vi "OceanOptics_TriggerPlayground_2.vi"() -> ()   [LabVIEW 2016]
uses:
  Maya2000 Typedefs/Maya2000 basic info.ctl
  <vilib>/Platform/TimedLoop/XDataNode/timing_clust.ctl
  <vilib>/Platform/TimedLoop/XDataNode/nitl_modes.ctl
  <vilib>/Platform/TimedLoop/XDataNode/wakeup.ctl
  C:/Program Files/Ocean Optics/OmniDriver/OOI_HOME/NETOmniDriver-NET40.dll
  Program Files/Ocean Optics/OmniDriver/OOI_HOME/NETOmniDriver-NET40.dll
  <vilib>/platform/TimedLoop/XDataNode/XDataNode.xnode
  <vilib>/Platform/TimedLoop/XDataNode/XDNodeRunTimeDep.lvlib
panel:
  out "spectrum":cluster{"Y":dbl[], "Y":dbl[]}[](graph)
  out "getExternalTriggerMode":i32
  in  "Trigger mode":i32
  out "isEnableBuffer":i32
  out "getBufferCapacity":i32
  in  "setBufferCoapacity":i32
  out "isFeatureSupportedDataBuffer":i16
  in  "clear":bool
  out "error Loop":errorcluster caption="error out"
  out "getExternalTriggerDelayIncrement":i32
  out "read":bool
  out "getBufferCapacity in Loop":i32
  out "getNumberOfElements before readout":i32
  out "status":bool
  out "error out":errorcluster
  out "this maya":T1={"This instruments index"=0, "Name+SerialNumber"="MayaPro2000:MAYP111403", "Number Dark pixels"=8, "NumberOfPixels\nper spectrum"=2068, "NumberOf Maya2000 instrm."=2, "MaximumIntegrationTime\n[us]"=1600000000, "MinimumIntegrationTime\n[us]"=7200}
  in  "stop":bool
  in  "integration time [us]":i32=100000
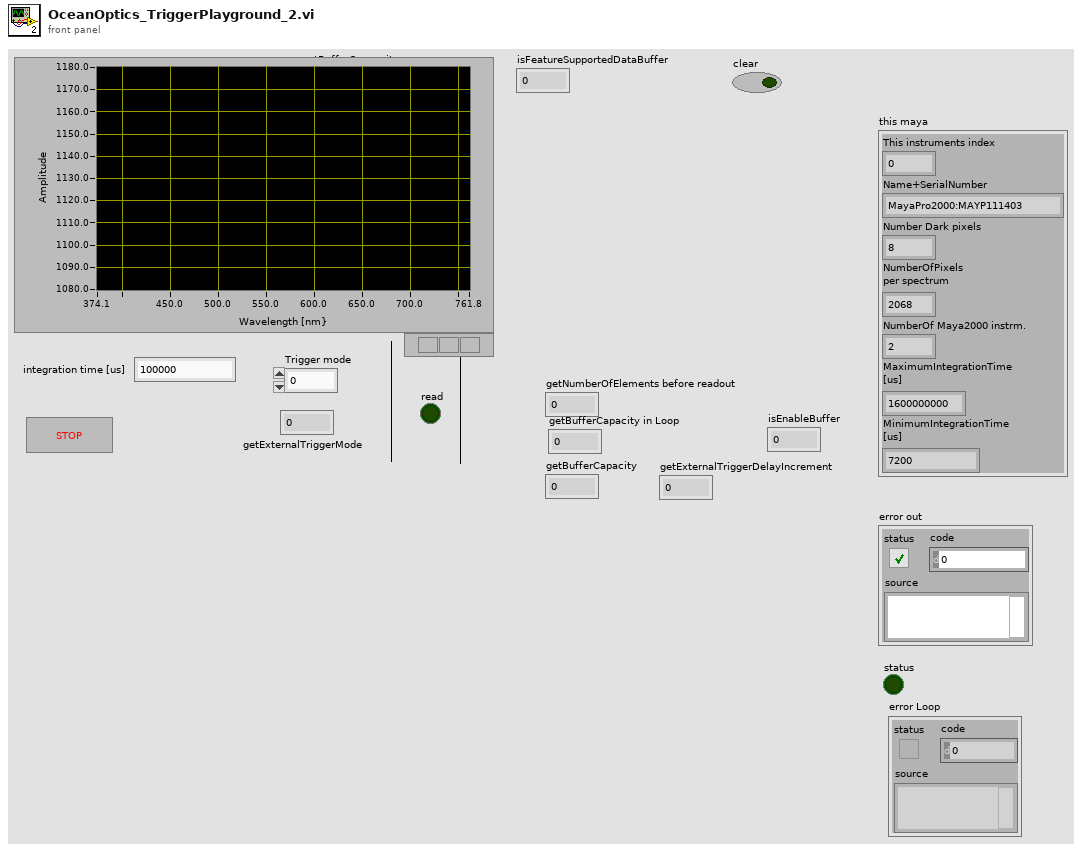
[diagram p1: front panel]
types:
  T1 = typedef "Maya2000 basic info.ctl" = cluster{"This instruments index":i32, "Name+SerialNumber":string, "Number Dark pixels":i32, "NumberOfPixels\nper spectrum":i32, "NumberOf Maya2000 instrm.":i32, "MaximumIntegrationTime\n[us]":i32, "MinimumIntegrationTime\n[us]":i32}
  T2 = typedef "XDNodeRunTimeDep.lvlib/timing_clust.ctl" = cluster{"Expected End [f-1]":u64, "Actual End [f-1]":u64, "Finished Late? [f-1]":bool, "Expected End [i-1]":u64, "Actual End [i-1]":u64, "Finished Late? [i-1]":bool, "Expected Start [i]":u64, "Actual Start [i]":u64, "Expected Start [f]":u64, "Actual Start [f]":u64, "Source Name":string, "Structure Name":string, "Period":i64, "Deadline":i64, "Offset":i64, "Start":i64, "Priority":i32, "Timeout":i32, "Mode":T3, "Wakeup Reason":T4, "Error":errorcluster, "Source Type":string, "Secondary Source Type":string, "Global End Time":u64, "Global Start Time":u64, "Frame Duration":u64, "Iteration Duration":u64, "Assigned CPU":i32, "I/O Scan Engine Mode":u32}
  T3 = typedef "XDNodeRunTimeDep.lvlib/nitl_modes.ctl" = enum32{"No Change", "Process missed periods, maintain original phase", "Discard missed periods, maintain original phase", "Process missed periods, ignore original phase", "Discard missed periods, ignore original phase"}
  T4 = typedef "XDNodeRunTimeDep.lvlib/wakeup.ctl" = enum32{"Normal", "Aborted", "Asynchronous wakeup", "Timing source error", "Timed loop error", "Timeout"}
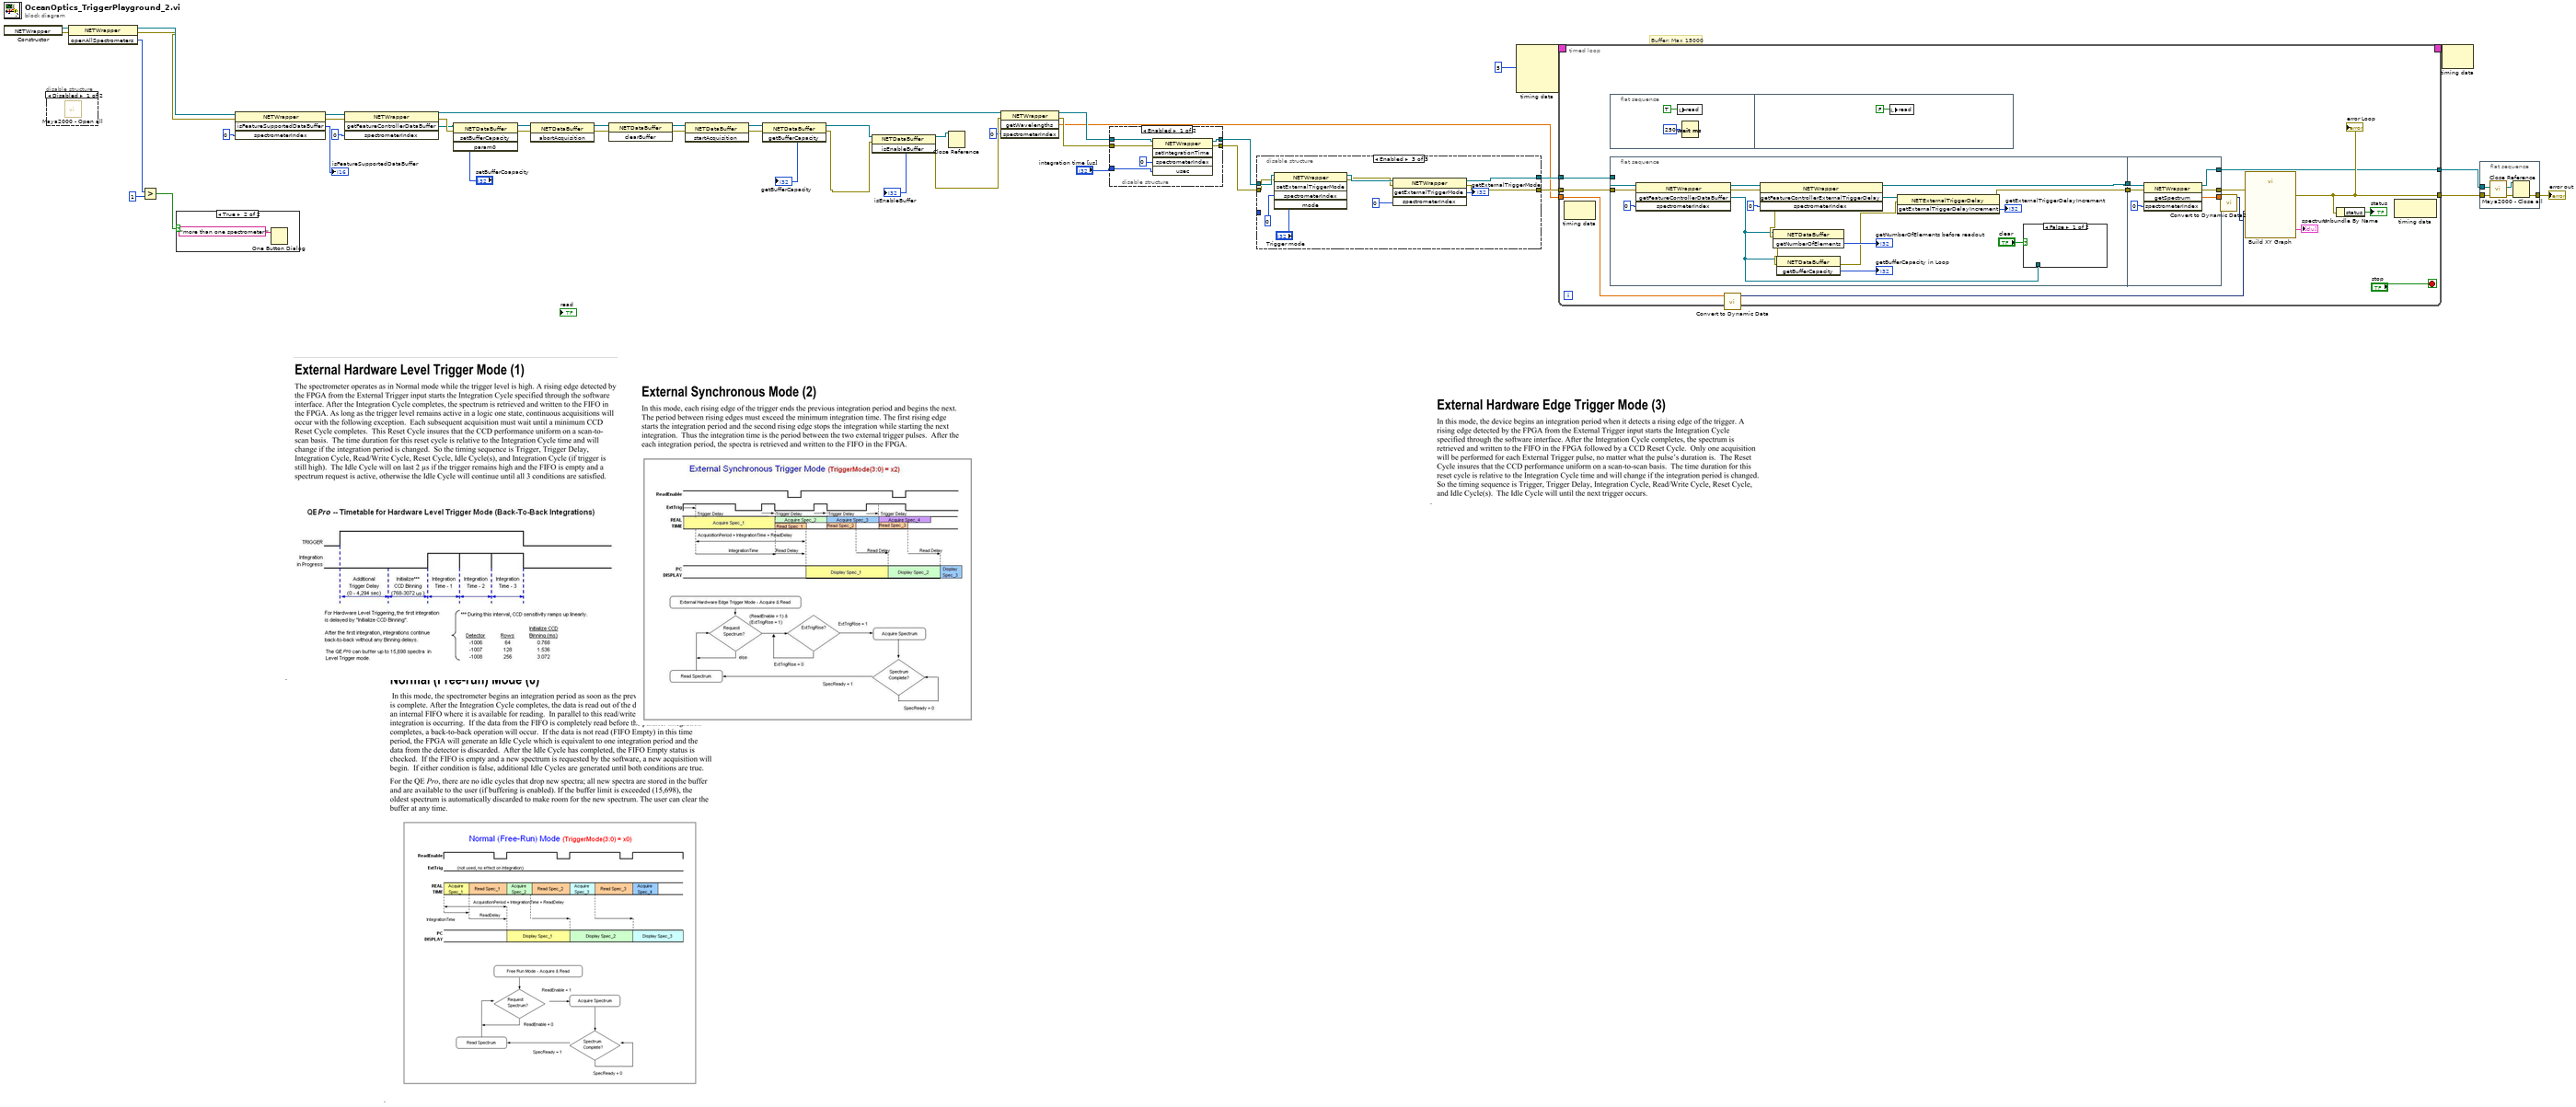
[diagram p0: block diagram]
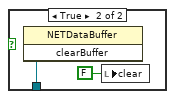
[diagram p3: hidden frame]
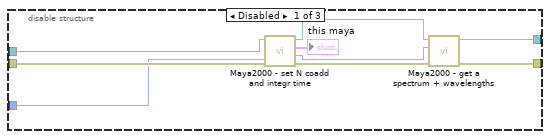
[diagram p4: hidden frame]
diagram:
  # "Buffer: Max 15000"
  n1 = constructor class="NETWrapper"() -> (reference out=w17:refnum<k24>, error out=w16:errorcluster)  [unwired: 3 in, 1 out]
  n2 = disable-structure shown="Disabled" {
    frame Disabled {
      n3 = call "Maya2000 - Open all.vi"() -> ()  [unwired: 9 in, 3 out]
    }
    frame Enabled {
    }
  }
  n4 = invoke class="NETWrapper" method="openAllSpectrometers"(reference=w17, error in=w16) -> (reference out=w15:refnum<k24>, error out=w14:errorcluster, "openAllSpectrometers"=w12:i32)  [unwired: 1 in]
  n5 = Greater?(x=w12, y=1) -> (0:w13:bool)
  n6 = case shown="True" w13 {
    frame False {
    }
    frame True {
      n7 = One Button Dialog(message="more than one spectrometer!") -> ()  [unwired: 1 in, 1 out]
    }
  }
  n8 = invoke class="NETWrapper" method="isFeatureSupportedDataBuffer"(reference=w15, error in=w14, "spectrometerIndex"=0) -> (reference out=w34:refnum<k24>, error out=w33:errorcluster, "isFeatureSupportedDataBuffer"=→"isFeatureSupportedDataBuffer":i16)  [unwired: 1 in, 1 out]
  n9 = invoke class="NETWrapper" method="getFeatureControllerDataBuffer"(reference=w34, error in=w33, "spectrometerIndex"=0) -> (reference out=w9:refnum<k24>, error out=w37:errorcluster, "getFeatureControllerDataBuffer"=w10:refnum<k24>)  [unwired: 1 in, 1 out]
  n10 = invoke class="NETDataBuffer" method="setBufferCapacity"(reference=w10, error in=w37, "param0"="setBufferCoapacity") -> (reference out=w22:refnum<k24>, error out=w31:errorcluster)  [unwired: 1 in, 2 out]
  n11 = invoke class="NETDataBuffer" method="abortAcquisition"(reference=w22, error in=w31) -> (reference out=w29:refnum<k24>, error out=w28:errorcluster)  [unwired: 1 in, 1 out]
  n12 = invoke class="NETDataBuffer" method="clearBuffer"(reference=w29, error in=w28) -> (reference out=w27:refnum<k24>, error out=w26:errorcluster)  [unwired: 1 in, 1 out]
  n13 = invoke class="NETDataBuffer" method="startAcquisition"(reference=w27, error in=w26) -> (reference out=w25:refnum<k24>, error out=w24:errorcluster)  [unwired: 1 in, 1 out]
  n14 = invoke class="NETDataBuffer" method="getBufferCapacity"(reference=w25, error in=w24) -> (reference out=w21:refnum<k24>, error out=w20:errorcluster, "getBufferCapacity"=→"getBufferCapacity":i32)  [unwired: 1 in]
  n15 = invoke class="NETDataBuffer" method="isEnableBuffer"(reference=w21, error in=w20) -> (reference out=w18:refnum<k24>, error out=w8:errorcluster, "isEnableBuffer"=→"isEnableBuffer":i16)  [unwired: 1 in]
  n16 = Close Reference(reference=w18) -> ()  [unwired: 1 in, 1 out]
  n17 = invoke class="NETWrapper" method="getWavelengths"(reference=w9, error in=w8, "spectrometerIndex"=0) -> (reference out=w5:refnum<k24>, error out=w2:errorcluster, "getWavelengths"=w1:dbl[])  [unwired: 1 in, 1 out]
  n18 = disable-structure shown="Enabled" {
    disable-tunnel: [w51 _] -> w4
    disable-tunnel: w5 -> [w50 _]
    disable-tunnel: "integration time [us]" -> [w49 _]
    disable-tunnel: [w48 _] -> w3
    disable-tunnel: w2 -> [w47 _]
    frame Enabled {
      n19 = invoke class="NETWrapper" method="setIntegrationTime"(reference=w50, error in=w47, "spectrometerIndex"=0 ("mode"), "usec"=w49) -> (reference out=w51:refnum<k24>, error out=w48:errorcluster)  [unwired: 1 in, 3 out]
    }
    frame Disabled {
    }
  }
  n20 = disable-structure shown="Enabled" {
    disable-tunnel: w4 -> [w63 _ w72]
    disable-tunnel: w3 -> [w61 _ w65]
    disable-tunnel: [w56 _ w70] -> w41
    disable-tunnel: [w54 _ w68] -> w42
    disable-tunnel: _ -> [w53 _ _]
    frame Disabled {
      n21 = call "Maya2000 - set N coadd and integr time.vi"("Intgration time\n[us]"=w53, "error in (no error)"=w61, ".NET Refnum in"=w63) -> ("error out"=w58:errorcluster, "This instruments index"=w55:i32, "This Maya´\nbasic info"=→"this maya":T1, ".NET Refnum out"=w59:refnum<k24>, "numberOfScans\nToAverage"=w60:u32, "Maya2000 basic values"=w62:T1[])  [unwired: 3 in]
      n22 = call "Maya2000 - get a spectrum + wavelengths.vi"("error in (no error)"=w58, "This instrments index"=w55, ".NET Refnum in"=w59) -> ("error out"=w54:errorcluster, "Wavelengths"=w57:dbl[], ".NET Refnum out"=w56:refnum<k24>)  [unwired: 3 in, 3 out]
    }
    frame Disabled {
    }
    frame Enabled {
      n23 = invoke class="NETWrapper" method="setExternalTriggerMode"(reference=w72, error in=w65, "spectrometerIndex"=0, "mode"="Trigger mode") -> (reference out=w71:refnum<k24>, error out=w69:errorcluster)  [unwired: 1 in, 3 out]
      n24 = invoke class="NETWrapper" method="getExternalTriggerMode"(reference=w71, error in=w69, "spectrometerIndex"=0) -> (reference out=w70:refnum<k24>, error out=w68:errorcluster, "getExternalTriggerMode"=→"getExternalTriggerMode":i32)  [unwired: 1 in, 1 out]
    }
  }
  n25 = node-c288(i64 5 ("Period")) -> (w40:T2)  [unwired: 3 in]
  n26 = timed-loop {
    tunnel: [w84] -> w44
    tunnel: [w77] -> w45
    tunnel: w1 -> [w83]
    tunnel: w41 -> [w80]
    tunnel: w42 -> [w81]
    timing: w40 -> [_]
    timing-out: [_] -> w39
    stop <- "stop" stop-if-true
    n27 = node-c288() -> ()  [unwired: 1 in, 1 out]
    n28 = flat-sequence {
      frame #0 {
        n29 = local write "read"(TRUE ("read")) -> ()
        n30 = Wait (ms)(milliseconds to wait=u32 250) -> ()  [unwired: 1 out]
      }
      frame #1 {
        n31 = local write "read"(FALSE ("read")) -> ()
      }
    }
    n32 = flat-sequence {
      tunnel: w80 -> [w102]
      tunnel: w81 -> [w97]
      tunnel: [w91] -> w79
      tunnel: [w95] -> w78
      tunnel: [w111] -> w77
      tunnel: [w108] -> w76
      tunnel: w79 -> [w109]
      tunnel: w78 -> [w107]
      tunnel: [w110] -> w75
      frame #0 {
        n33 = invoke class="NETWrapper" method="getFeatureControllerDataBuffer"(reference=w102, error in=w97, "spectrometerIndex"=0) -> (error out=w96:errorcluster, "getFeatureControllerDataBuffer"=w90:refnum<k24>)  [unwired: 1 in, 2 out]
        n34 = invoke class="NETWrapper" method="getFeatureControllerExternalTriggerDelay"(reference=w102, error in=w96, "spectrometerIndex"=0) -> (reference out=w95:refnum<k24>, error out=w94:errorcluster, "getFeatureControllerExternalTriggerDelay"=w103:refnum<k24>)  [unwired: 1 in, 1 out]
        n35 = invoke class="NETDataBuffer" method="getNumberOfElements"(reference=w90, error in=w94) -> (error out=w93:errorcluster, "getNumberOfElements"=→"getNumberOfElements before readout":i32)  [unwired: 1 in, 1 out]
        n36 = invoke class="NETDataBuffer" method="getBufferCapacity"(reference=w90, error in=w93) -> (error out=w92:errorcluster, "getBufferCapacity"=→"getBufferCapacity in Loop":i32)  [unwired: 1 in, 1 out]
        n37 = invoke class="NETExternalTriggerDelay" method="getExternalTriggerDelayIncrement"(reference=w103, error in=w92) -> (error out=w91:errorcluster, "getExternalTriggerDelayIncrement"=→"getExternalTriggerDelayIncrement":i32)  [unwired: 1 in, 1 out]
        n38 = case shown="False" "clear" {
          tunnel: w90 -> [_ w106]
          frame False {
          }
          frame True {
            n39 = invoke class="NETDataBuffer" method="clearBuffer"(reference=w106) -> ()  [unwired: 2 in, 3 out]
            n40 = local write "clear"(FALSE ("clear")) -> ()
          }
        }
      }
      frame #1 {
        n41 = invoke class="NETWrapper" method="getSpectrum"(reference=w107, error in=w109, "spectrometerIndex"=0) -> (reference out=w111:refnum<k24>, error out=w108:errorcluster, "getSpectrum"=w110:dbl[])  [unwired: 1 in, 1 out]
      }
    }
    n42 = call "Convert to Dynamic Data"("Array"=w83) -> ("Dynamic Data Type"=w87:dynamicdata)  [unwired: 3 in]
    n43 = call "Convert to Dynamic Data2"("Array"=w75) -> ("Dynamic Data Type"=w86:dynamicdata)  [unwired: 3 in]
    n44 = call "Build XY Graph"("error in (no error)"=w76, "Y Input"=w86, "X Input"=w87) -> ("error out"=w84:errorcluster, "XY Graph"=→"spectrum":cluster{"X":dbl[], "Y":dbl[]}[])  [unwired: 7 in]
    "error Loop" <- w84
    n45 = Unbundle By Name(w84) -> ("status"=→"status":bool)
    n46 = node-c288() -> ()  [unwired: 1 in, 1 out]
  }
  n47 = node-c288(w39) -> ()  [unwired: 1 out]
  n48 = flat-sequence {
    tunnel: w45 -> [w122]
    tunnel: w44 -> [w121]
    tunnel: [w120] -> w43
    frame #0 {
      n49 = call "Maya2000 - Close all.vi"("error in (no error)"=w121, "Maya reference in"=w122) -> ("error out"=w119:errorcluster, ".NET Refnum out"=w118:refnum<k24>)  [unwired: 8 in]
      n50 = Close Reference(reference=w118, error in (no error)=w119) -> (error out=w120:errorcluster)
    }
  }
  "error out" <- w43
